vi "LC DB Read_Control.vi"(8 "error in (no error)":errorcluster caption="Error In", 11 "Table Name":string) -> (0 "error out":errorcluster caption="Error Out", 3 "Data":string[][](array[string]))   [LabVIEW 2020]
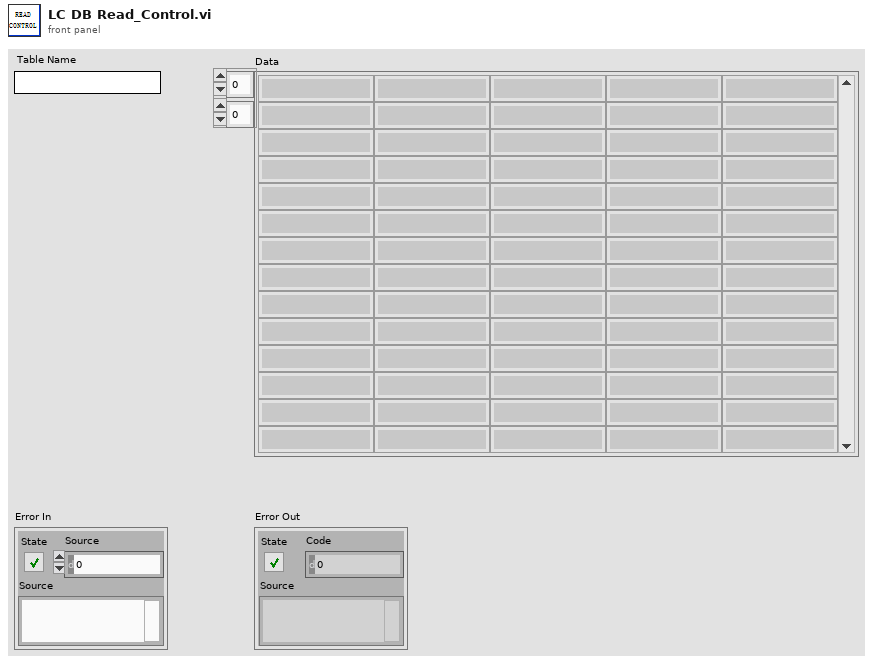
[diagram p1: front panel]
types:
  T1 = typedef "NI_Database_API.lvlib/Conn ObjectReference.ctl" = refnum<k1>
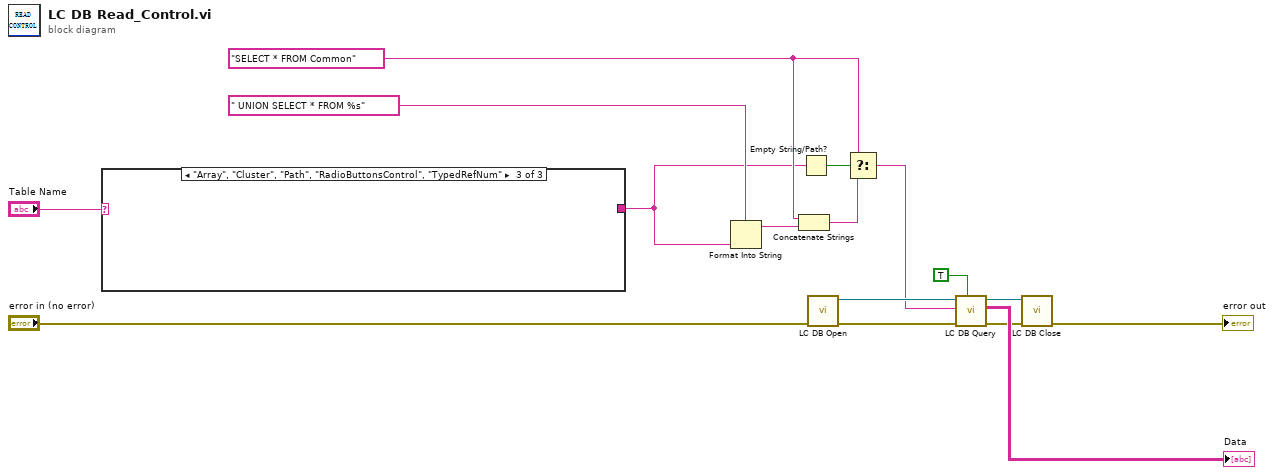
[diagram p0: block diagram]
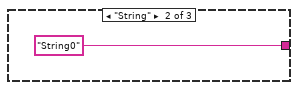
[diagram p3: hidden frame]
diagram:
  w5 = "SELECT * FROM Common" ("SQL query")
  n1 = case shown="\"Array\", \"Cluster\", \"Path\", \"RadioButtonsControl\", \"TypedRefNum\"" "Table Name" {
    selector: "Table Name" -> [w17 _ _]
    tunnel: [w17 "String0" _] -> w1
    frame "eee", Default {
    }
    frame "String" {
    }
    frame "Array", "Cluster", "Path", "RadioButtonsControl", "TypedRefNum" {
    }
  }
  n2 = Format Into String(format string=" UNION SELECT * FROM %s" ("SQL query"), w1) -> (resulting string=w4:string)  [unwired: 2 in, 1 out]
  n3 = Concatenate Strings(w5, w4) -> (w3:string)
  n4 = Empty String/Path?(string/path=w1) -> (empty?=w6:bool)
  n5 = call "LC DB Open.vi"("error in (no error)"="error in (no error)") -> ("error out"=w11:errorcluster, "DB Ref Out"=w12:T1)  [unwired: 9 in]
  n6 = Select(t=w5, s=w6, f=w3) -> (s? t:f=w2:string)
  n7 = call "LC DB Query.vi"("Read?"=TRUE, "error in (no error)"=w11, "SQL query"=w2, "DB Ref In"=w12) -> ("error out"=w9:errorcluster, "Data"=→"Data":string[][], "DB Ref Out"=w10:T1)  [unwired: 5 in]
  n8 = call "LC DB Close.vi"("error in (no error)"=w9, "DB Ref In"=w10) -> ("error out"=→"error out":errorcluster)  [unwired: 9 in]
